vi "Mercury_GoToField.vi"(8 "error in":errorcluster, 10 "put into persistent mode after reaching target field?":bool, 11 "Mercury Targets":T1={"Target Field (T)"=0.1, "Target Field Rate (T/min)"=0.1} {"Target Field (T)" format="%.4g"; "Target Field Rate (T/min)" format="%.4g"}) -> (0 "error out":errorcluster)   [LabVIEW 2013]
doc: "Use this VI to remotely interact with the Oxford Mercury power supply through \"Oxford-1820-Main.vi\", which MUST also be running."
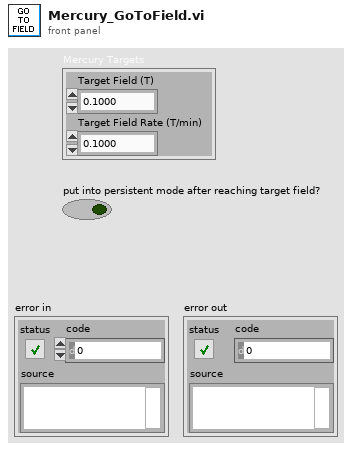
[diagram p1: front panel]
types:
  T1 = cluster{"Target Field (T)":dbl, "Target Field Rate (T/min)":dbl}
  T2 = cluster{"Hold":bool, "Clamp":bool, "To Set":bool, "To Zero":bool, "Send to IPS":bool, "PS Heat":bool, "Lambda":bool}
  T3 = cluster{"Magnet Field":dbl, "PS Field":dbl, "Target Field":dbl, "Target Field Rate":dbl, "Voltage":dbl, "Current":dbl, "Switch":bool}
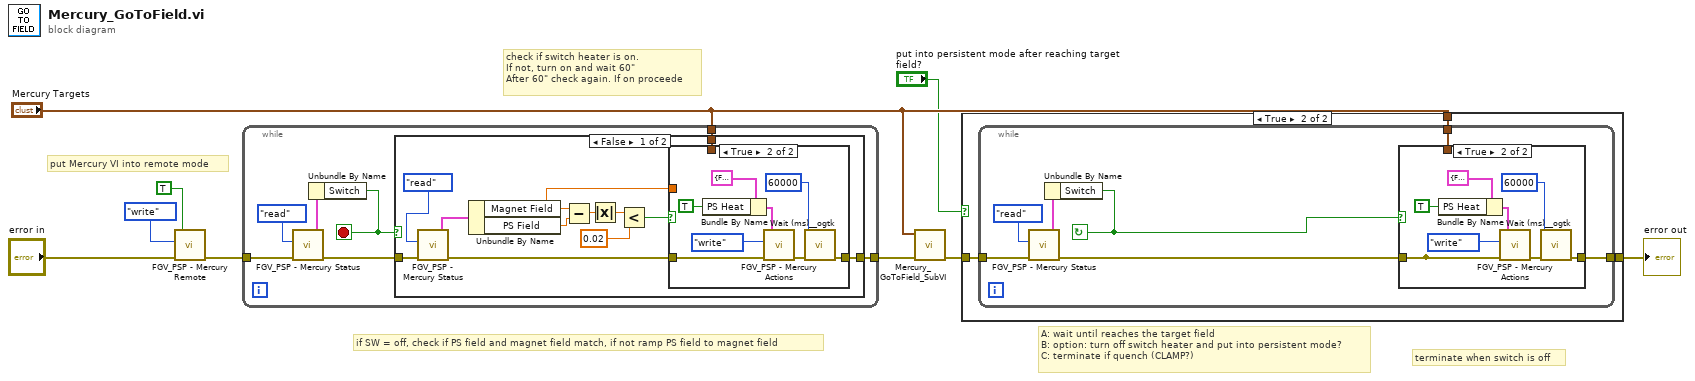
[diagram p0: block diagram]
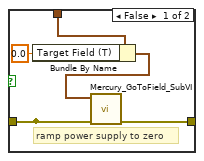
[diagram p3: hidden frame]
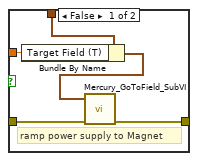
[diagram p4: hidden frame]
diagram:
  # "terminate when switch is off"
  # "A: wait until reaches the target field\nB: option: turn off switch heater and put into persistent mode?\nC: terminate if quench (CLAMP?)"
  # "if SW = off, check if PS field and magnet field match, if not ramp PS field to magnet field"
  # "check if switch heater is on.\nIf not, turn on and wait 60\"\nAfter 60\" check again. If on proceede"
  # "put Mercury VI into remote mode"
  n1 = call "FGV_PSP - Mercury Remote.vi"("error in"="error in", "Function"=enum16{"write", "read"}."write", "Mercury Remote"=TRUE) -> ("error out"=w8:errorcluster)  [unwired: 3 in, 1 out]
  n2 = while {
    tunnel: [w13] -> w9
    tunnel: w8 -> [w12]
    tunnel: "Mercury Targets" -> [w10]
    stop <- w14 stop-if-true
    n3 = call "FGV_PSP - Mercury Status.vi"("error in"=w12, "Function"=enum16{"write", "read"}."read") -> ("error out"=w15:errorcluster, "status"=w16:T3)  [unwired: 4 in]
    n4 = Unbundle By Name(w16) -> ("Switch"=w14:bool)
    n5 = case shown="False" w14 {
      tunnel: w15 -> [w27 w42]
      tunnel: [w28 w42] -> w13
      tunnel: w10 -> [w19 _]
      frame False {
        n6 = call "FGV_PSP - Mercury Status.vi"("error in"=w27, "Function"=enum16{"write", "read"}."read") -> ("error out"=w25:errorcluster, "status"=w26:T3)  [unwired: 4 in]
        n7 = Unbundle By Name(w26) -> ("Magnet Field"=w18:dbl, "PS Field"=w24:dbl)
        n8 = Subtract(x=w18, y=w24) -> (x-y=w23:dbl)
        n9 = Absolute Value(x=w23) -> (abs(x)=w22:dbl)
        n10 = Less?(x=w22, y=0.02) -> (x < y?=w20:bool)
        n11 = case shown="True" w20 {
          tunnel: [w32 w36] -> w28
          tunnel: w25 -> [w33 w34]
          tunnel: w19 -> [w31 _]
          tunnel: w18 -> [w30 _]
          frame False {
            # "ramp power supply to Magnet"
            n12 = Bundle By Name(cluster=w31, "Target Field (T)"=w30) -> (w29:T1)
            n13 = call "Mercury_GoToField_SubVI.vi"("error in (no error)"=w33, "Mercury Targets"=w29) -> ("error out"=w32:errorcluster)  [unwired: 9 in]
          }
          frame True {
            n14 = Bundle By Name(cluster=T2 {"Hold"=FALSE, "Clamp"=FALSE, "To Set"=FALSE, "To Zero"=FALSE, "Send to IPS"=FALSE, "PS Heat"=FALSE, "Lambda"=FALSE} ("mercury actions"), "PS Heat"=TRUE ("Send to IPS")) -> (w38:T2)
            n15 = call "FGV_PSP - Mercury Actions.vi"("error in"=w34, "Function"=enum16{"write", "read"}."write", "mercury actions"=w38) -> ("error out"=w37:errorcluster)  [unwired: 3 in, 1 out]
            n16 = call <userlib>:"Wait (ms)__ogtk.vi"("error in (no error)"=w37, "milliseconds to wait"=u32 60000) -> ("error out"=w36:errorcluster)  [unwired: 8 in, 1 out]
          }
        }
      }
      frame True {
      }
    }
  }
  n17 = call "Mercury_GoToField_SubVI.vi"("error in (no error)"=w9, "Mercury Targets"="Mercury Targets") -> ("error out"=w4:errorcluster)  [unwired: 9 in]
  n18 = case shown="True" "put into persistent mode after reaching target field?" {
    tunnel: w4 -> [w43 w46]
    tunnel: "Mercury Targets" -> [_ w45]
    tunnel: [w43 w44] -> w2
    frame False {
    }
    frame True {
      n19 = while {
        tunnel: [w52] -> w44
        tunnel: w46 -> [w51]
        tunnel: w45 -> [w49]
        stop <- w48 continue-if-true
        n20 = call "FGV_PSP - Mercury Status.vi"("error in"=w51, "Function"=enum16{"write", "read"}."read") -> ("error out"=w47:errorcluster, "status"=w53:T3)  [unwired: 4 in]
        n21 = Unbundle By Name(w53) -> ("Switch"=w48:bool)
        n22 = case shown="True" w48 {
          tunnel: [w58 w61] -> w52
          tunnel: [w54 w59] -> _
          tunnel: w49 -> [w57 _]
          tunnel: w47 -> [w54 w59]
          frame False {
            # "ramp power supply to zero"
            n23 = Bundle By Name(cluster=w57, "Target Field (T)"=0.0) -> (w56:T1)
            n24 = call "Mercury_GoToField_SubVI.vi"("error in (no error)"=w54, "Mercury Targets"=w56) -> ("error out"=w58:errorcluster)  [unwired: 9 in]
          }
          frame True {
            n25 = Bundle By Name(cluster=T2 {"Hold"=FALSE, "Clamp"=FALSE, "To Set"=FALSE, "To Zero"=FALSE, "Send to IPS"=FALSE, "PS Heat"=FALSE, "Lambda"=FALSE} ("mercury actions"), "PS Heat"=TRUE ("Send to IPS")) -> (w63:T2)
            n26 = call "FGV_PSP - Mercury Actions.vi"("error in"=w59, "Function"=enum16{"write", "read"}."write", "mercury actions"=w63) -> ("error out"=w62:errorcluster)  [unwired: 3 in, 1 out]
            n27 = call <userlib>:"Wait (ms)__ogtk.vi"("error in (no error)"=w62, "milliseconds to wait"=u32 60000) -> ("error out"=w61:errorcluster)  [unwired: 8 in, 1 out]
          }
        }
      }
    }
  }
  "error out" <- w2
